vi "PH_4_Pos_Selector.set GUI Elements.vi"(0 "i ref in":refnum<vi>, 5 "error in (no error)":errorcluster) -> (14 "i ref out":refnum<vi>, 19 "error out":errorcluster)   [LabVIEW 2014, in "PH_4_Pos_Selector.lvlib"]
doc: "This VI sets GUI tip strips and the visibility of GUI elements."
uses:
  PH_4_Pos_Selector.lvlib
  PH_Common/PH_Common.lvlib
  PH_AxisGUI_BaseClass/PH_AxisGUI_BaseClass.lvlib
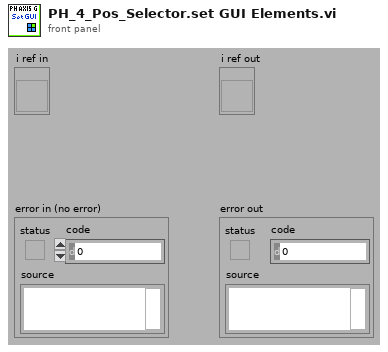
[diagram p1: front panel]
types:
  T1 = typedef "PH_4_Pos_Selector.lvlib/PH_4_Pos_Selector.i attribute.ctl" = cluster{"GUI Refs":cluster{"Position I":refnum<vi>, "Position II":refnum<vi>, "Position III":refnum<vi>, "Position IV":refnum<vi>, "rel. Mode?":refnum<vi>, "Define Selector":refnum<vi>}, "Current Position":T2, "Service ID Position":i32, "Position Array":T3[], "Description Array":string[], "relative Mode":bool, "Wanted Define Selector Position":string}
  T2 = typedef "PH_4_Pos_Selector.lvlib/PH_4_Pos_Selector.Position Selector.ctl" = u16
  T3 = typedef "PH_4_Pos_Selector.lvlib/PH_4_Pos_Selector.Position.ctl" = cluster{"Axis 1":dbl, "Axis 2":dbl}
  T4 = typedef "PH_AxisGUI_BaseClass.lvlib/PH_AxisGUI_BaseClass.i attribute.ctl" = cluster{"Axes":T5[]}
  T5 = typedef "PH_AxisGUI_BaseClass.lvlib/PH_AxisGUI_BaseClass.Axis Attributes.ctl" = cluster{"Axis GUI Refs":T6, "Address":T7, "Name":string, "Label \"Back\"":string, "Labell \"Forth\"":string, "Moving?":bool}
  T6 = typedef "PH_AxisGUI_BaseClass.lvlib/PH_AxisGUI_BaseClass.Axis GUI Refs.ctl" = cluster{"Back":refnum<vi>, "Forth":refnum<vi>, "Status":refnum<vi>, "Target":refnum<vi>, "Address":refnum<vi>, "Status Bar":refnum<vi>, "Settings":refnum<vi>, "Activity":refnum<vi>, "Clear Error":refnum<vi>}
  T7 = typedef "PH_Stepmotor_BaseClass.lvlib/PH_Stepmotor_BaseClass.Axis Address.ctl" = cluster{"Instance":string, "Motor Nr":i32}
  T8 = typedef "PH_Stepmotor_BaseClass.lvlib/PH_Stepmotor_BaseClass.Axis Settings.ctl" = cluster{"Sign change":bool, "Width":dbl, "Calibration":dbl, "Unit":string, "Motor Type":T9, "Unit Width":string, "Unit CF":string}
  T9 = typedef "PH_Stepmotor_BaseClass.lvlib/PH_Stepmotor_BaseClass.Motor Type.ctl" = enum16{"Unspecific", "OWIS 49.120.2633", "OWIS 49.060.1033", "OWIS 43.040.2558", "Diamond Motion 2200 series", "OWIS 49.120.266B.MV6", "Calorimeter", "Linear Stage 1", "MICOS VT-80", "MICOS VT-80 S", "Standa Rotstage nt0.95A", "PUF RA 320.200", "PUF RA 800.200", "PUF RA 800.400", "PUF RA 400.50", "1324.nn.800.50", "1324.n9c.800.50", "1324.nn.320.200", "1324.nn.400.200", "1324.nn.800.200", "1324.nn.400.50", "1324.8c9c.800.50", "1324.8c9c.400.200"}
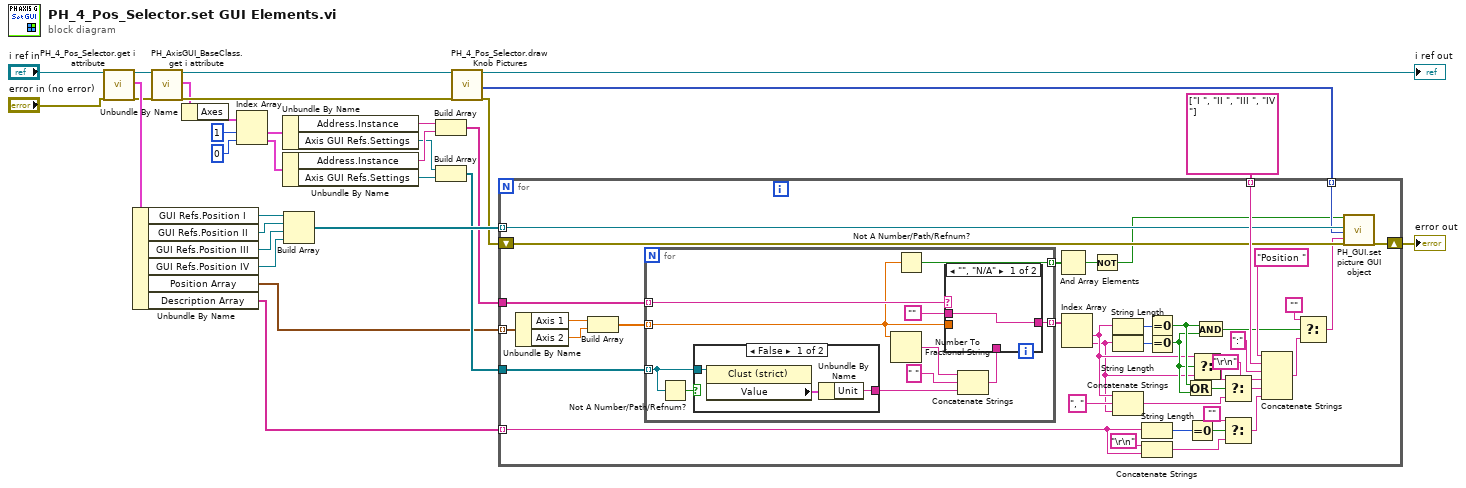
[diagram p0: block diagram]
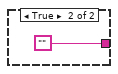
[diagram p2: hidden frame]
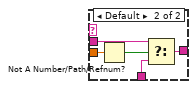
[diagram p3: hidden frame]
diagram:
  n1 = call "PH_4_Pos_Selector.get i attribute.vi"("i ref in"="i ref in", "error in (no error)"="error in (no error)") -> ("i ref out"=w24:refnum<vi>, "i attribute"=w31:T1, "error out"=w23:errorcluster)  [unwired: 15 in]
  n2 = Unbundle By Name(w31) -> ("GUI Refs.Position I"=w30:refnum<vi>, "GUI Refs.Position II"=w29:refnum<vi>, "GUI Refs.Position III"=w28:refnum<vi>, "GUI Refs.Position IV"=w27:refnum<vi>, "Position Array"=w4:T3[], "Description Array"=w3:string[])
  n3 = call "PH_AxisGUI_BaseClass.get i attribute.vi"("i ref in"=w24, "error in (no error)"=w23) -> ("i ref out"=w20:refnum<vi>, "i attribute"=w17:T4, "error out"=w21:errorcluster)  [unwired: 15 in]
  n4 = Unbundle By Name(w17) -> ("Axes"=w16:T5[])
  n5 = Index Array(array=w16, index #1=1 ("index"), index #2=0 ("index")) -> (element #1=w13:T5, element #2=w11:T5)
  n6 = Unbundle By Name(w13) -> ("Address.Instance"=w12:string, "Axis GUI Refs.Settings"=w9:refnum<vi>)
  n7 = Unbundle By Name(w11) -> ("Address.Instance"=w10:string, "Axis GUI Refs.Settings"=w8:refnum<vi>)
  n8 = Build Array(w30, w29, w28, w27) -> (w26:refnum<vi>[])
  n9 = Build Array(w12, w10) -> (w22:string[])
  n10 = Build Array(w9, w8) -> (w5:refnum<vi>[])
  n11 = call "PH_4_Pos_Selector.draw Knob Pictures.vi"("i ref in"=w20, "error in"=w21) -> ("i ref out"=→"i ref out":refnum<vi>, "Picture Array"=w18:picture[], "error out"=w7:errorcluster)  [unwired: 15 in]
  n12 = for {
    tunnel: w26 -> [w41] mode=indexing
    tunnel: w4 -> [w71] mode=indexing
    tunnel: string[] ["I ", "II ", "III ", "IV "] -> [w70] mode=indexing
    tunnel: w3 -> [w69] mode=indexing
    tunnel: w22 -> [w38]
    tunnel: w18 -> [w37] mode=indexing
    shift-right: [w33] -> w6
    shift-left: w7 -> [w40]
    tunnel: w5 -> [w32]
    n13 = Unbundle By Name(w71) -> ("Axis 1"=w50:dbl, "Axis 2"=w49:dbl)
    n14 = Build Array(w50, w49) -> (w68:dbl[])
    n15 = for {
      tunnel: w68 -> [w76] mode=indexing
      tunnel: [w78] -> w65 mode=indexing
      tunnel: w38 -> [w77] mode=indexing
      tunnel: [w75] -> w36 mode=indexing
      tunnel: w32 -> [w72] mode=indexing
      n16 = Not A Number/Path/Refnum?(number/path/refnum=w72) -> (NaN/Path/Refnum?=w73:bool)
      n17 = case shown="False" w73 {
        tunnel: w72 -> [w85 _]
        tunnel: [w83 ""] -> w74
        frame False {
          n18 = property class="Clust (strict)"(reference=w85) -> ("Value"=w84:T8)  [unwired: 1 in, 2 out]
          n19 = Unbundle By Name(w84) -> ("Unit"=w83:string)
        }
        frame True {
        }
      }
      n20 = Number To Fractional String(number=w76) -> (F-format string=w81:string)  [unwired: 3 in]
      n21 = Not A Number/Path/Refnum?(number/path/refnum=w76) -> (NaN/Path/Refnum?=w75:bool)
      n22 = Concatenate Strings(w81, " " ("string"), w74) -> (w80:string)
      n23 = case shown="\"\", \"N/A\"" w77 {
        tunnel: w76 -> [_ w92]
        tunnel: "" -> [w87 w91]
        tunnel: w80 -> [_ w90]
        tunnel: [w87 w89] -> w78
        frame "", "N/A" {
        }
        frame Default {
          n24 = Not A Number/Path/Refnum?(number/path/refnum=w92) -> (NaN/Path/Refnum?=w88:bool)
          n25 = Select(t=w91, s=w88, f=w90) -> (s? t:f=w89:string)
        }
      }
    }
    n26 = And Array Elements(Boolean array=w36) -> (logical AND=w35:bool)
    n27 = Index Array(array=w65) -> (element #1=w53:string, element #2=w52:string)  [unwired: 2 in]
    n28 = Not(x=w35) -> (.not. x?=w34:bool)
    n29 = String Length(string=w53) -> (length=w64:i32)
    n30 = String Length(string=w52) -> (length=w63:i32)
    n31 = Concatenate Strings(w53, ", " ("string"), w52) -> (w55:string)
    n32 = String Length(string=w69) -> (length=w47:i32)
    n33 = Concatenate Strings("\r\n", w69) -> (w42:string)
    n34 = Equal To 0?(x=w64) -> (x = 0?=w60:bool)
    n35 = Equal To 0?(x=w63) -> (x = 0?=w54:bool)
    n36 = Or(x=w60, y=w54) -> (x .or. y?=w59:bool)
    n37 = Equal To 0?(x=w47) -> (x = 0?=w46:bool)
    n38 = Select(t=w53, s=w54, f=w52) -> (s? t:f=w51:string)
    n39 = And(x=w60, y=w54) -> (x .and. y?=w62:bool)
    n40 = Select(t=w51, s=w59, f=w55) -> (s? t:f=w57:string)
    n41 = Select(t="", s=w46, f=w42) -> (s? t:f=w44:string)
    n42 = Concatenate Strings("Position ", w70, ":" ("string"), "\r\n", w57, w44) -> (w58:string)
    n43 = Select(t="", s=w62, f=w58) -> (s? t:f=w39:string)
    n44 = call "PH_GUI.set picture GUI object.vi"("Visible (true)"=w34, "CtlRef"=w41, "Picture"=w37, "Tip Strip (\"\")"=w39, "error in (no error)"=w40) -> ("error out"=w33:errorcluster)  [unwired: 14 in]
  }
  "error out" <- w6
